vi "Update Item.vi"(8 "error in (no error)":errorcluster, 9 "New Item":refnum<class "Data Item.lvclass">, 10 "Tag":string, 11 "Tree Manager in":refnum<class "Tree Manager.lvclass">) -> (0 "error out":errorcluster, 3 "Tree Manager out":refnum<class "Tree Manager.lvclass">)   [LabVIEW 2020, in "VILab.lvlib" / "Tree Manager.lvclass"]
uses:
  Tree Manager.lvclass
  Data Item/Data Item.lvclass
  Tree Manager.lvclass/Tree Manager.ctl
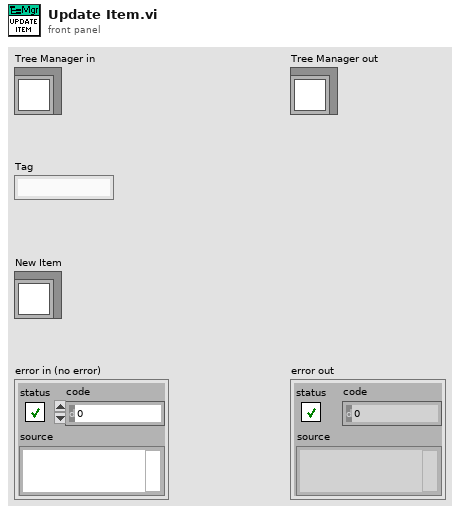
[diagram p1: front panel]
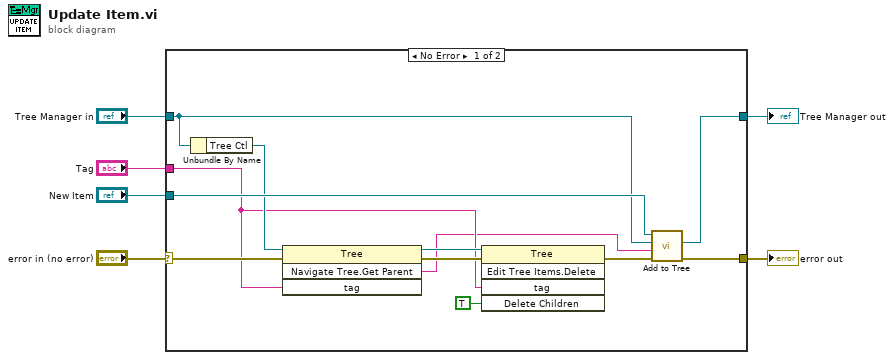
[diagram p0: block diagram]
diagram:
  n1 = case shown="No Error" "error in (no error)" {
    selector: "error in (no error)" -> [w14 w20]
    tunnel: [w10 w20] -> w5
    tunnel: [w11 w19] -> w3
    tunnel: "Tree Manager in" -> [w8 w19]
    tunnel: "Tag" -> [w9 _]
    tunnel: "New Item" -> [w17 _]
    frame No Error {
      n2 = Unbundle By Name(w8) -> ("Tree Ctl"=w15:refnum<vi>)
      n3 = invoke class="Tree" method="Navigate Tree.Get Parent"(reference=w15, error in=w14, "tag"=w9) -> (reference out=w13:refnum<vi>, error out=w12:errorcluster, "Navigate Tree:Get Parent"=w7:string)  [unwired: 1 in, 1 out]
      n4 = invoke on="Delete" class="Tree" method="Edit Tree Items.Delete"(reference=w13, error in=w12, "tag"=w9, "Delete Children"=TRUE ("Delete Children?")) -> (error out=w16:errorcluster)  [unwired: 1 in, 4 out]
      n5 = call-dynamic "Add to Tree.vi"("error in (no error)"=w16, "Parent Tag"=w7, "Tree Manager in"=w8, "Data Item in"=w17) -> ("error out"=w10:errorcluster, "Tree Manager out"=w11:refnum<class "Tree Manager.lvclass">)  [unwired: 5 in, 1 out]
    }
    frame Error {
    }
  }
  "error out" <- w5
  "Tree Manager out" <- w3
